vi "queueexample.vi"() -> ()   [LabVIEW 2015]
panel:
  out "Waveform Chart":dbl(graph)
  in  "stop":bool
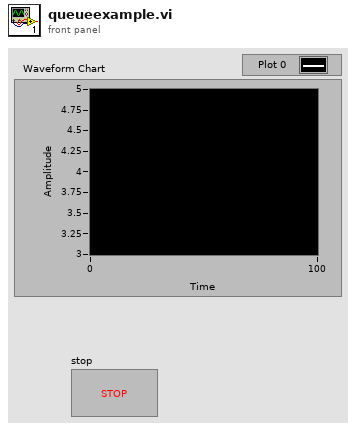
[diagram p1: front panel]
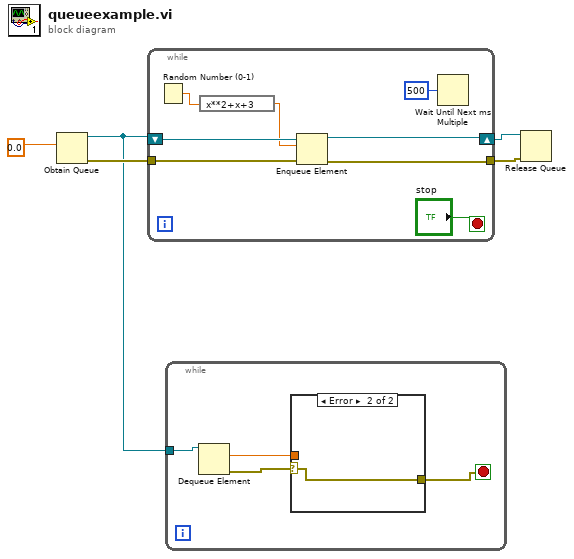
[diagram p0: block diagram]
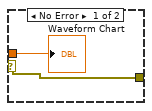
[diagram p2: hidden frame]
diagram:
  n1 = Obtain Queue(element data type=0.0) -> (queue out=w1:refnum<queue>, error out=w3:errorcluster)  [unwired: 4 in, 1 out]
  n2 = while {
    tunnel: [w12] -> w4
    tunnel: w3 -> [w13]
    shift-right: [w10] -> w2
    shift-left: w1 -> [w11]
    stop <- "stop" stop-if-true
    n3 = Random Number (0-1)() -> (number: 0 to 1=w7:dbl)
    n4 = expression code="x**2+x+3"(w7) -> (w6:dbl)
    n5 = Enqueue Element(queue=w11, element=w6, error in (no error)=w13) -> (queue out=w10:refnum<queue>, error out=w12:errorcluster)  [unwired: 1 in, 1 out]
    n6 = Wait Until Next ms Multiple(millisecond multiple=u32 500) -> ()  [unwired: 1 out]
  }
  n7 = while {
    tunnel: w1 -> [w17]
    stop <- w15 stop-if-true
    n8 = Dequeue Element(queue=w17) -> (element=w14:dbl, error out=w16:errorcluster)  [unwired: 2 in, 2 out]
    n9 = case shown="Error" w16 {
      selector: w16 -> [w19 w20]
      tunnel: [w19 w20] -> w15
      tunnel: w14 -> [w18 _]
      frame No Error {
        "Waveform Chart" <- w18
      }
      frame Error {
      }
    }
  }
  n10 = Release Queue(queue=w2, error in (no error)=w4) -> ()  [unwired: 1 in, 3 out]
